vi "Shift Direction Plane.vi"(10 "Direction":T1, 11 "Direction Plane":T1[][](array[typedef])) -> (3 "Direction Plane Out":T1[][](array[typedef]))   [LabVIEW 2023]
uses:
  RB ENUM_Position ID.ctl
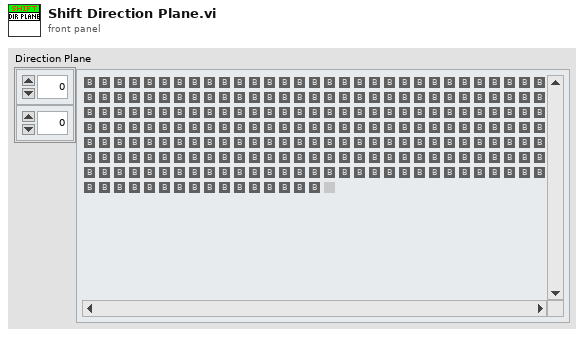
[diagram p1: front panel]
types:
  T1 = typedef "RB ENUM_Position ID.ctl" = enum32{"Blank", "Wall", "UP", "Down", "Left", "Right", "Two", "Three", "Four", "Spot"}
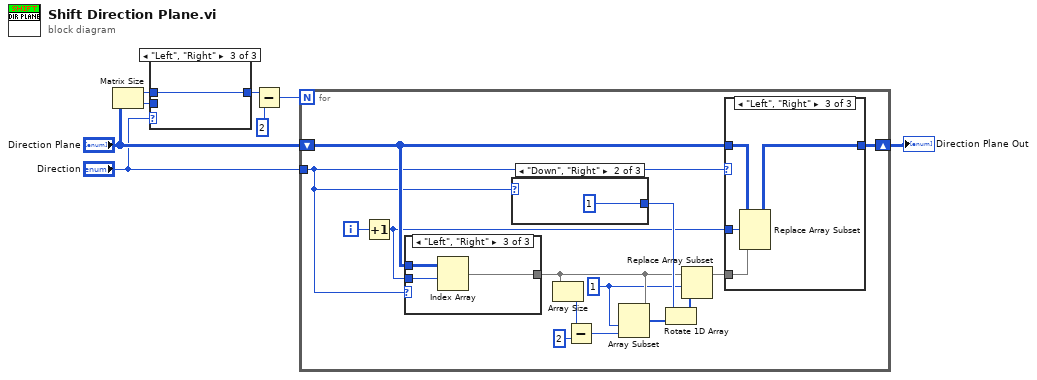
[diagram p0: block diagram]
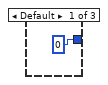
[diagram p2: hidden frame]
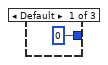
[diagram p4: hidden frame]
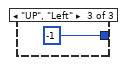
[diagram p5: hidden frame]
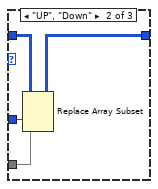
[diagram p7: hidden frame]
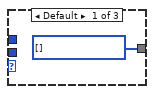
[diagram p8: hidden frame]
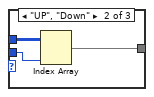
[diagram p9: hidden frame]
diagram:
  n1 = Matrix Size(0:"Direction Plane") -> (1:w3:i32, 2:w1:i32)
  n2 = case shown="\"Left\", \"Right\"" "Direction" {
    tunnel: [0 w10 w11] -> w2
    tunnel: w3 -> [_ _ w11]
    tunnel: w1 -> [_ w10 _]
    frame Default {
    }
    frame "UP", "Down" {
    }
    frame "Left", "Right" {
    }
  }
  n3 = Subtract(x=w2, y=2) -> (x-y=w5:i32)
  n4 = for {
    N: w5 -> [_]
    shift-right: [w21] -> w7
    shift-left: "Direction Plane" -> [w24]
    tunnel: "Direction" -> [w23]
    i -> [w25]
    w12 = 1 ("index")
    n5 = Increment(x=w25) -> (x+1=w20:i32)
    n6 = case shown="\"Left\", \"Right\"" w23 {
      tunnel: w24 -> [_ w41 w44]
      tunnel: w20 -> [_ w40 w43]
      tunnel: [w38 w39 w42] -> w15
      frame Default {
        w38 = T1[] [] items=["Blank", "Wall", "UP", "Down", "Left", "Right", "Two", "Three", "Four", "Spot"] ("Direction Plane")
      }
      frame "UP", "Down" {
        n7 = Index Array(array=w41, index (col)=w40) -> (element=w39:T1[])  [unwired: 1 in]
      }
      frame "Left", "Right" {
        n8 = Index Array(array=w44, index (row)=w43) -> (element=w42:T1[])  [unwired: 1 in]
      }
    }
    n9 = case shown="\"Down\", \"Right\"" w23 {
      tunnel: [0 1 -1] -> w22
      frame Default {
      }
      frame "Down", "Right" {
      }
      frame "UP", "Left" {
      }
    }
    n10 = Array Size(array=w15) -> (size(s)=w19:i32)
    n11 = Subtract(x=w19, y=2) -> (x-y=w16:i32)
    n12 = Array Subset(array=w15, index=w12, length=w16) -> (w17:T1[])
    n13 = Rotate 1D Array(1:w17, 2:w22) -> (0:w13:T1[])
    n14 = Replace Array Subset(array=w15, new element=w13, index=w12) -> (w14:T1[])
    n15 = case shown="\"Left\", \"Right\"" w23 {
      tunnel: w24 -> [w29 w33 w37]
      tunnel: [w29 w32 w36] -> w21
      tunnel: w20 -> [_ w31 w35]
      tunnel: w14 -> [_ w30 w34]
      frame Default {
      }
      frame "UP", "Down" {
        n16 = Replace Array Subset(array=w33, new element=w30, index (col)=w31) -> (w32:T1[][])  [unwired: 1 in]
      }
      frame "Left", "Right" {
        n17 = Replace Array Subset(array=w37, new element=w34, index (row)=w35) -> (w36:T1[][])  [unwired: 1 in]
      }
    }
  }
  "Direction Plane Out" <- w7
